vi "Load Param Database (Core).vi"(8 "error in":errorcluster, 9 "hw db path in":path, 10 "parm db path in":path, 11 "Node Ptr":u64) -> (0 "error out":errorcluster)   [LabVIEW 2020, in "Ballard 1553 System Explorer.lvlib"]
uses:
  Ballard 1553 System Explorer.lvlib
  <vilib>/NI VeriStand/Custom Device API/Custom Device API.lvlib
  <vilib>/NI VeriStand/Custom Device API/Get Item Property (Path).vi
  <vilib>/NI VeriStand/Custom Device Tools/Custom Device Utility Library/Custom Device Utility Library.lvlib
  <vilib>/NI VeriStand/Custom Device API/Set Item Property (Path).vi
  <vilib>/NI VeriStand/Custom Device API/Set Item Property (String).vi
  Shared/Controls and Global/Global.vi
  Shared/Ballard 1553 Shared.lvlib
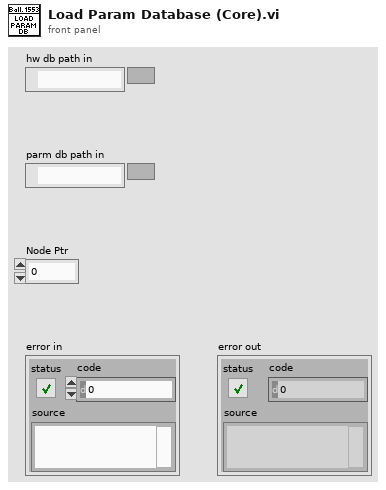
[diagram p1: front panel]
types:
  T1 = typedef "Custom Device API.lvlib/Custom Device Item Ref.ctl" = u64
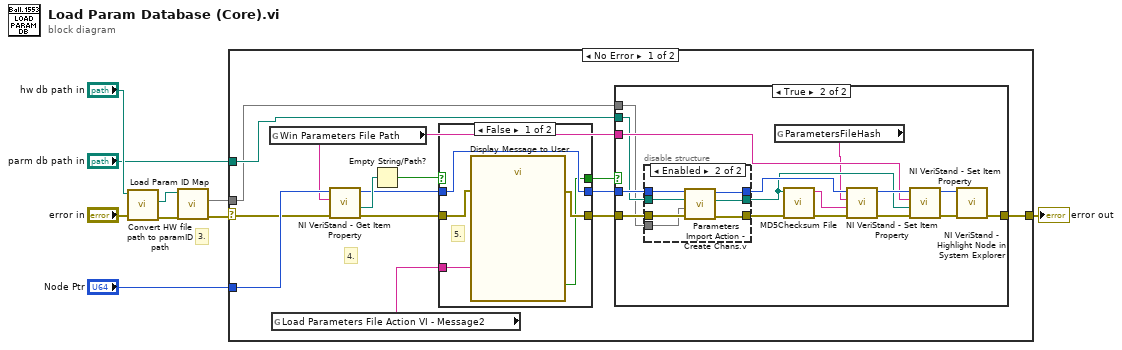
[diagram p0: block diagram]
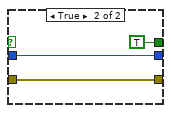
[diagram p2: hidden frame]
diagram:
  # "3."
  n1 = call "Convert HW file path to paramID path.vi"("error in (no error)"="error in", "Hw File In"="hw db path in") -> ("error out"=w7:errorcluster, "Param Id File out"=w6:path)  [unwired: 7 in, 1 out]
  n2 = call "Load Param ID Map.vi"("error in (no error)"=w7, "Param Id File in"=w6) -> ("error out"=w8:errorcluster, "Param ID map"=w9:map{i32, string})  [unwired: 7 in, 1 out]
  n3 = case shown="No Error" w8 {
    selector: w8 -> [w20 w59]
    tunnel: [w23 w59] -> w1
    tunnel: "Node Ptr" -> [w22 _]
    tunnel: "parm db path in" -> [w13 _]
    tunnel: w9 -> [w10 _]
    frame No Error {
      # "4."
      n4 = global read "Global.vi" "Win Parameters File Path"() -> (w12:string)
      n5 = global read "Global.vi" "Load Parameters File Action VI - Message2"() -> (w11:string)
      n6 = call-poly <vilib>:"NI VeriStand - Get Item Property.vi"("error in (no error)"=w20, "Property Name"=w12, "Item Ref in"=w22) -> ("error out"=w18:errorcluster, "Value"=w21:path, "Item Ref out"=w17:T1)  [unwired: 5 in, 1 out]
      n7 = Empty String/Path?(string/path=w21) -> (empty?=w19:bool)
      n8 = case shown="False" w19 {
        tunnel: w18 -> [w27 w30]
        tunnel: w17 -> [w28 w29]
        tunnel: [w25 TRUE] -> w16
        tunnel: [w26 w30] -> w15
        tunnel: [w28 w29] -> w14
        tunnel: w11 -> [w24 _]
        frame False {
          # "5."
          n9 = call "Display Message to User"("error in (no error)"=w27, "Message"=w24) -> ("error out"=w26:errorcluster, "OK"=w25:bool)  [unwired: 8 in]
        }
        frame True {
        }
      }
      n10 = case shown="True" w16 {
        tunnel: [w32 w48] -> w23
        tunnel: w12 -> [_ w41]
        tunnel: w15 -> [w32 w39]
        tunnel: w14 -> [_ w40]
        tunnel: w13 -> [_ w36]
        tunnel: w10 -> [_ w33]
        frame False {
        }
        frame True {
          n11 = disable-structure shown="Enabled" {
            disable-tunnel: w40 -> [w49 w56]
            disable-tunnel: w39 -> [w51 w58]
            disable-tunnel: [w49 w53] -> w38
            disable-tunnel: [w51 w55] -> w37
            disable-tunnel: w36 -> [w50 w57]
            disable-tunnel: [w50 w54] -> w35
            disable-tunnel: w33 -> [_ w52]
            frame Disabled {
            }
            frame Enabled {
              n12 = call "Parameters Import Action - Create Chans.v.vi"("error in (no error)"=w58, "Param ID map"=w52, "selected path"=w57, "Item Ref in"=w56) -> ("error out"=w55:errorcluster, "selected path out"=w54:path, "Item Ref out"=w53:T1)  [unwired: 5 in]
            }
          }
          n13 = global read "Global.vi" "ParametersFileHash"() -> (w34:string)
          n14 = call <vilib>:"MD5Checksum File.vi"("error in (no error)"=w37, "Path"=w35) -> ("error out"=w43:errorcluster, "MD5 message-digest"=w42:string)  [unwired: 8 in]
          n15 = call-poly <vilib>:"NI VeriStand - Set Item Property.vi"("error in (no error)"=w43, "Value"=w42, "Property Name"=w34, "Item Ref in"=w38) -> ("error out"=w44:errorcluster, "Item Ref out"=w45:T1)  [unwired: 5 in, 1 out]
          n16 = call-poly <vilib>:"NI VeriStand - Set Item Property.vi"("error in (no error)"=w44, "Value"=w35, "Property Name"=w41, "Item Ref in"=w45) -> ("error out"=w47:errorcluster, "Item Ref out"=w46:T1)  [unwired: 5 in, 1 out]
          n17 = call <vilib>:"NI VeriStand - Highlight Node in System Explorer.vi"("error in (no error)"=w47, "Item Ref in"=w46) -> ("error out"=w48:errorcluster)  [unwired: 8 in, 1 out]
        }
      }
    }
    frame Error {
    }
  }
  "error out" <- w1
